vi "Write Vehicle out of Position Ref.vi"(4 "Vehicle Out of Position Ref":refnum<vi>, 11 "Active Station View Definition in":refnum<class "Active Option View Definition.lvclass">) -> (3 "Active Station View Definition out":refnum<class "Active Option View Definition.lvclass">)   [LabVIEW 2019, in "Active Option View Definition.lvclass"]
uses:
  <vilib>/gpm_packages/@cs/Car-wash/Source/Active Station View Definition/Active Station View Definition/Active Option View Definition.lvclass
  <vilib>/gpm_packages/@cs/Car-wash/Source/Active Station View Definition/Active Station View Definition/Active Option View Definition.lvclass/Active Option View Definition.ctl
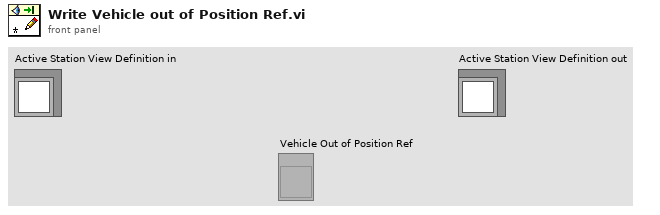
[diagram p1: front panel]
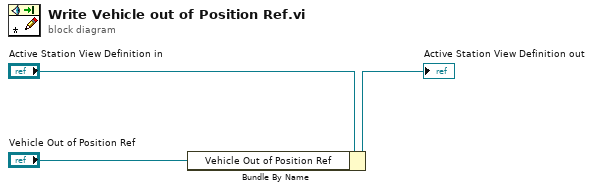
[diagram p0: block diagram]
diagram:
  n1 = Bundle By Name(cluster="Active Station View Definition in", "Vehicle Out of Position Ref"="Vehicle Out of Position Ref") -> (→"Active Station View Definition out":refnum<class "Active Option View Definition.lvclass">)
